vi "Fichier.vi"(11 "Nom de fichier":string) -> (0 "error out":errorcluster, 3 "Byte Stream File out":refnum<file>)   [LabVIEW 2014]
doc: "Create, or open a file"
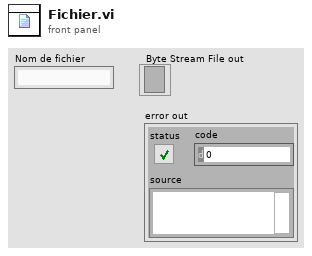
[diagram p1: front panel]
types:
  T1 = enum16{"open", "replace", "create", "open or create", "replace or create", "replace or create with confirmation"}
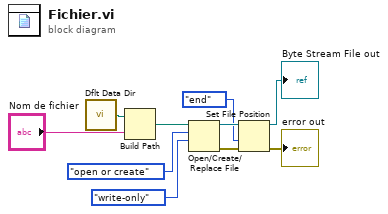
[diagram p0: block diagram]
diagram:
  n1 = call <vilib>:"Dflt Data Dir.vi"() -> ("App:Default Data Directory"=w7:path)
  n2 = Build Path(base path=w7, name or relative path="Nom de fichier") -> (appended path=w4:path)
  n3 = Open/Create/Replace File(file path (use dialog)=w4, operation (0:open)=T1."open or create", access (0:read/write)=enum16{"read/write", "read-only", "write-only"}."write-only") -> (refnum out=w10:refnum<file>, error out=w9:errorcluster)  [unwired: 1 in, 3 out]
  n4 = Set File Position(refnum=w10, from (0:start)=enum16{"start", "end", "current"}."end", error in=w9) -> (refnum out=→"Byte Stream File out":refnum<file>, error out=→"error out":errorcluster)  [unwired: 1 in]
